vi "Remove Constant Array.vi"(0 "Function String":string, 11 "error in (no error)":errorcluster) -> (4 "Replace Sub Function with variable":string, 6 "Sub Functions":string[](array[string]), 8 "Variables":string[](array[string]), 15 "error out":errorcluster)   [LabVIEW 2019]
panel:
  # "{1,2,3}\n{1,2,3},{4,5,6}\n{{1,2,3}{4,5,6}},{1,2}}"
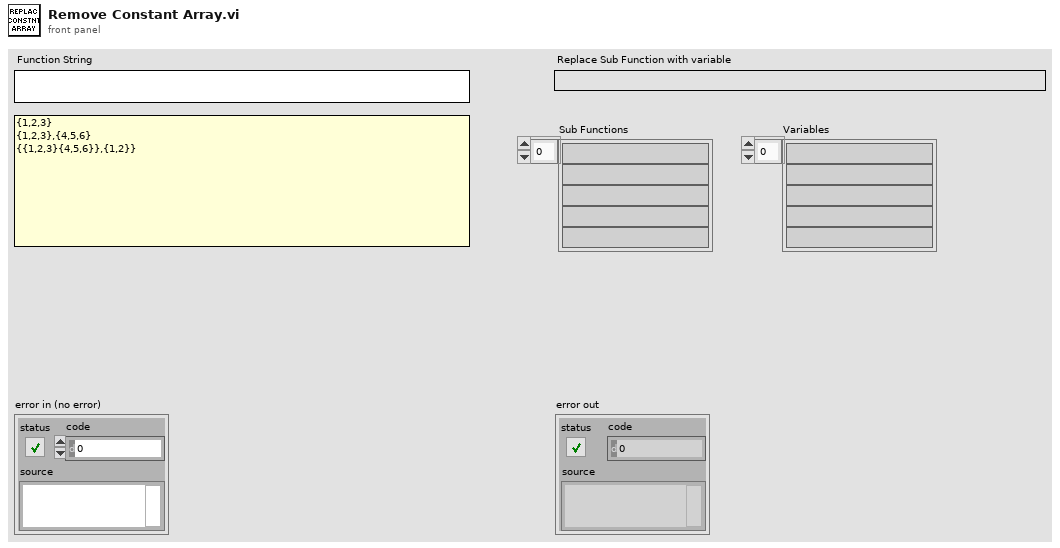
[diagram p1: front panel]
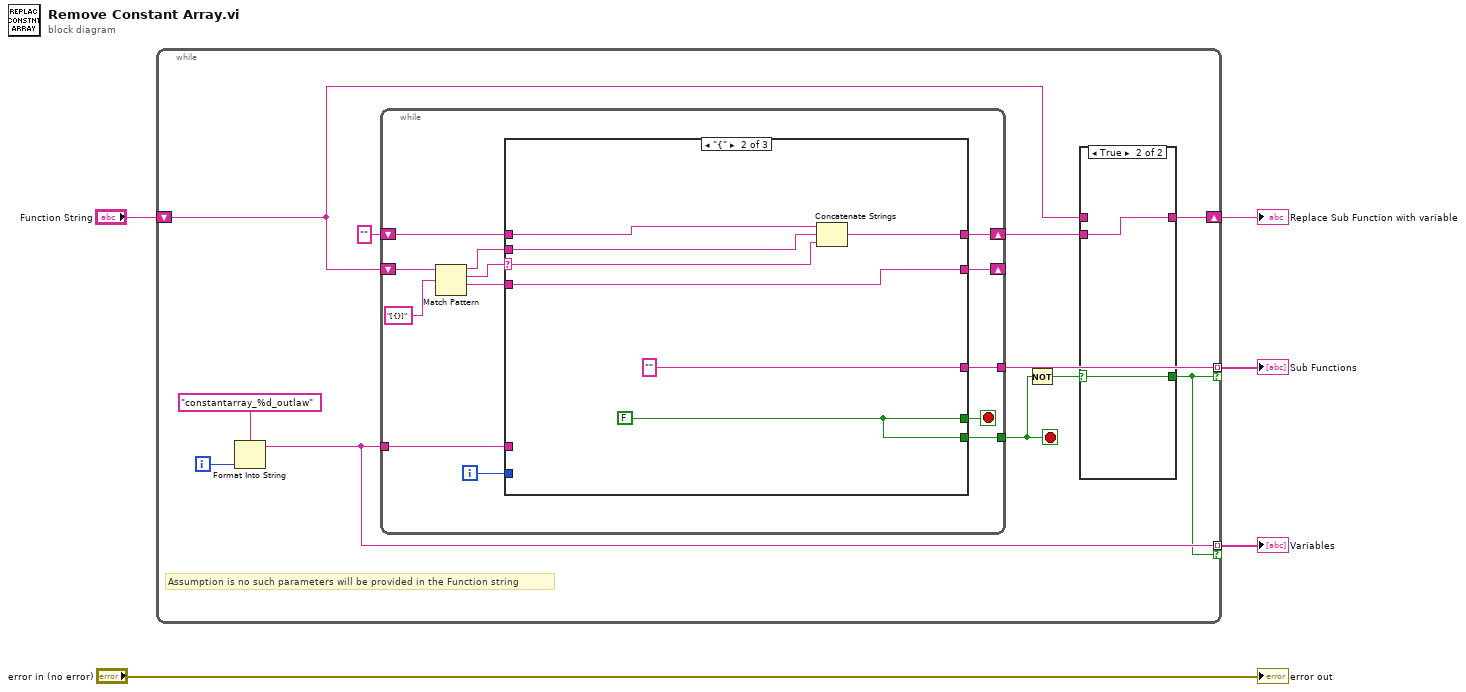
[diagram p0: block diagram]
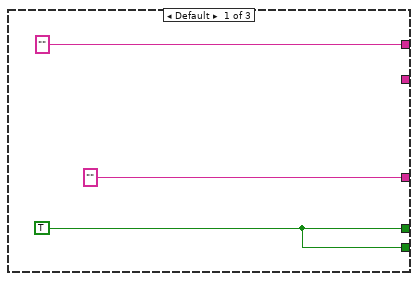
[diagram p3: hidden frame]
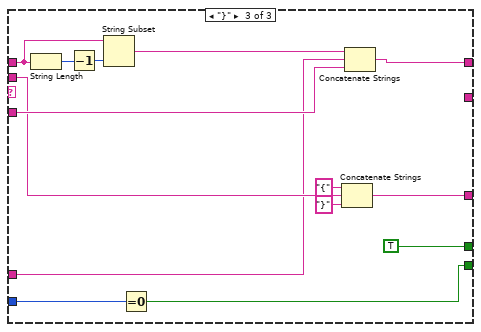
[diagram p4: hidden frame]
diagram:
  n1 = while {
    tunnel: [w16] -> w2 mode=indexing if=w7
    tunnel: [w8] -> w1 mode=indexing if=w7
    shift-right: [w13] -> w3
    shift-left: "Function String" -> [w12]
    i -> [w10]
    stop <- w15 stop-if-true
    # "Assumption is no such parameters will be provided in the Function string"
    n2 = Format Into String(format string="constantarray_%d_outlaw", w10) -> (resulting string=w8:string)  [unwired: 2 in, 1 out]
    n3 = while {
      tunnel: [w29] -> w15
      shift-right: [w26] -> _
      shift-left: w12 -> [w25]
      tunnel: [w24] -> w16
      shift-right: [w28] -> w11
      shift-left: "" ("Function String") -> [w23]
      tunnel: w8 -> [w22]
      i -> [w21]
      stop <- w30 stop-if-true
      n4 = Match Pattern(string=w25, regular expression="[{}]") -> (before substring=w31:string, match substring=w32:string, after substring=w27:string)  [unwired: 1 in, 1 out]
      n5 = case shown="\"{\"" w32 {
        selector: w32 -> [_ w40 _]
        tunnel: w31 -> [_ w37 w55]
        tunnel: ["" ("Function String") w39 w46] -> w28
        tunnel: [w36 w42 TRUE] -> w30
        tunnel: [w36 w42 w47] -> w29
        tunnel: w27 -> [_ w43 w56]
        tunnel: [_ w43 _] -> w26
        tunnel: ["" "" w54] -> w24
        tunnel: w23 -> [_ w38 w48]
        tunnel: w22 -> [_ _ w45]
        tunnel: w21 -> [_ _ w51]
        frame Default {
          w36 = TRUE
        }
        frame "{" {
          w42 = FALSE
          n6 = Concatenate Strings(w38, w37, w40) -> (w39:string)
        }
        frame "}" {
          n7 = String Length(string=w48) -> (length=w49:i32)
          n8 = Decrement(x=w49) -> (x-1=w50:i32)
          n9 = String Subset(string=w48, length (rest)=w50) -> (substring=w44:string)  [unwired: 1 in]
          n10 = Equal To 0?(x=w51) -> (x = 0?=w47:bool)
          n11 = Concatenate Strings("{" ("string"), w55, "}" ("string")) -> (w54:string)
          n12 = Concatenate Strings(w44, w45, w56) -> (w46:string)
        }
      }
    }
    n13 = Not(x=w15) -> (.not. x?=w14:bool)
    n14 = case shown="True" w14 {
      selector: w14 -> [w17 w20]
      tunnel: [w18 w19] -> w13
      tunnel: w12 -> [w18 _]
      tunnel: [w17 w20] -> w7
      tunnel: w11 -> [_ w19]
      frame False {
      }
      frame True {
      }
    }
  }
  "Replace Sub Function with variable" <- w3
  "Sub Functions" <- w2
  "Variables" <- w1
  "error out" <- "error in (no error)"
